vi "Adaptive Drain.vi"(0 "GEA2 Reference In":refnum<k24>, 1 "TC":dbl=1.2 format="%#_13g", 2 "H":dbl=5.0, 5 "BC":dbl=15.9 format="%#_13g", 7 "FC":dbl=-0.9 format="%#_13g", 9 "AD Timeout (s)":dbl=360.0 format="%#_13g", 11 "Error In":errorcluster, 12 "Pressure Threshold (Inchesx1000)":string="500") -> (3 "Actual Drain Time":dbl, 4 "GEA2 Reference Out":refnum<k24>, 6 "Pass/Fail?":bool, 10 "Report Text":string, 14 "Calculated Drain Time":dbl, 15 "Error Out":errorcluster)   [LabVIEW 2016, in "TLMB.lvlib"]
uses:
  Projects/TLMB.lvlib
  Q:/Common/DLLs/GEA3/GeaCommunication.dll
  Common/DLLs/GEA3/GeaCommunication.dll
  Common/LabVIEW GEA2 Toolkit/LabVIEW_GEA2_Toolkit.lvlibp/type defs/Source_Destination.ctl
  Common/LabVIEW GEA2 Toolkit/LabVIEW_GEA2_Toolkit.lvlibp/type defs/ERD Read Data In.ctl
  Common/LabVIEW GEA2 Toolkit/LabVIEW_GEA2_Toolkit.lvlibp/type defs/Data Type.ctl
  Common/LabVIEW GEA2 Toolkit/LabVIEW_GEA2_Toolkit.lvlibp
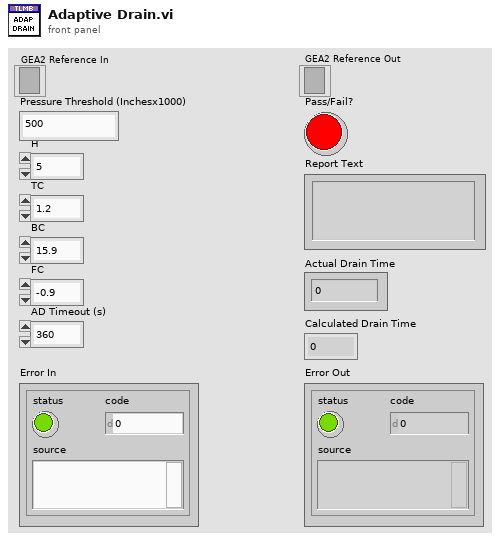
[diagram p1: front panel]
types:
  T1 = enum16{"EQ (==)", "NE (!=)", "GT (>)", "LT (<)", "GE (>=)", "LE (<=)", "GTLT(> <)", "GELE (>= <=)", "GELT (>= <)", "GTLE (> <=)", "LTGT (< >)", "LEGE (<= >=)", "LEGT (<= >)", "LTGE (< >=)", "No Comparison"}
  T2 = typedef "LabVIEW_GEA2_Toolkit.lvlibp/ERD Read Data In.ctl" = cluster{"ERD Number":u16, "Data Type":T3}
  T3 = typedef "LabVIEW_GEA2_Toolkit.lvlibp/Data Type.ctl" = enum16{"string", "boolean", "uint8_t", "uint16_t", "uint32_t", "uint64_t", "int8_t", "int16_t", "int32_t", "int64_t"}
  T4 = typedef "LabVIEW_GEA2_Toolkit.lvlibp/Source_Destination.ctl" = cluster{"Source":u8, "Destination":u8}
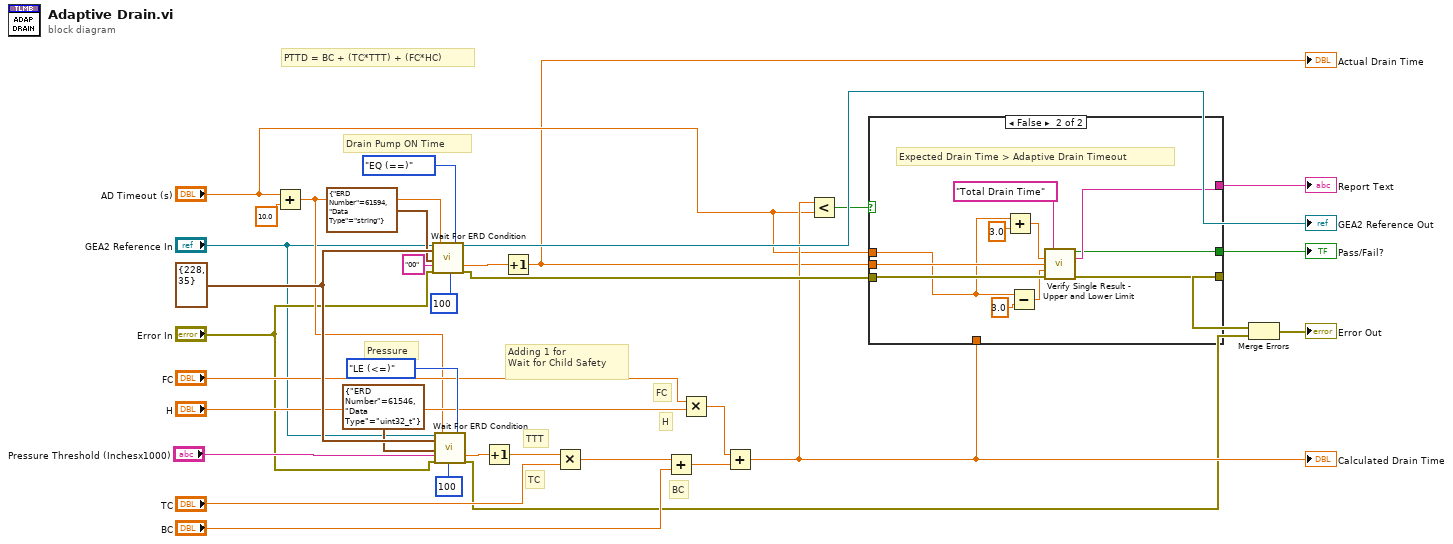
[diagram p0: block diagram]
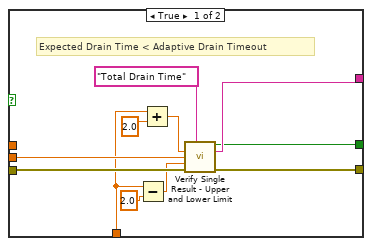
[diagram p2: hidden frame]
diagram:
  w34 = T4 {"Source"=228, "Destination"=35} ("GEA Inputs")
  # "Drain Pump ON Time"
  # "Pressure"
  # "Adding 1 for \nWait for Child Safety"
  # "H"
  # "FC"
  # "TTT"
  # "TC"
  # "BC"
  # "PTTD = BC + (TC*TTT) + (FC*HC)"
  n1 = Add(x="AD Timeout (s)", y=10.0) -> (x+y=w10:dbl)
  n2 = call "Wait For ERD Condition.vi"("GEA2 Reference In"="GEA2 Reference In", "GEA Inputs"=w34, "ERD Read Data"=T2 {"ERD Number"=61594, "Data Type"=enum."string"}, "Expected Low"="00", "Error In"="Error In", "Timeout (s)"=w10, "Loop Rate (ms)"=u32 100, "Comparison"=T1."EQ (==)") -> ("GEA2 Reference Out"=→"GEA2 Reference Out":refnum<k24>, "Execution Time"=w17:dbl, "Error Out"=w18:errorcluster)  [unwired: 7 in, 2 out]
  n3 = call "Wait For ERD Condition.vi"("GEA2 Reference In"="GEA2 Reference In", "GEA Inputs"=w34, "ERD Read Data"=T2 {"ERD Number"=61546, "Data Type"=enum."uint32_t"}, "Expected Low"="Pressure Threshold (Inchesx1000)", "Error In"="Error In", "Timeout (s)"=w10, "Loop Rate (ms)"=u32 100, "Comparison"=T1."LE (<=)") -> ("Execution Time"=w26:dbl, "Error Out"=w5:errorcluster)  [unwired: 7 in, 3 out]
  n4 = Increment(x=w26) -> (x+1=w23:dbl)
  n5 = Increment(x=w17) -> (x+1=w1:dbl)
  "Actual Drain Time" <- w1
  n6 = Multiply(x=w23, y="TC") -> (x*y=w22:dbl)
  n7 = Add(x=w22, y="BC") -> (x+y=w20:dbl)
  n8 = Multiply(x="FC", y="H") -> (x*y=w19:dbl)
  n9 = Add(x=w19, y=w20) -> (x+y=w9:dbl)
  "Calculated Drain Time" <- w9
  n10 = Less?(x=w9, y="AD Timeout (s)") -> (x < y?=w8:bool)
  n11 = case shown="False" w8 {
    tunnel: w1 -> [w45 w56]
    tunnel: w9 -> [w36 _]
    tunnel: w18 -> [w44 w55]
    tunnel: [w43 w54] -> w4
    tunnel: [w40 w51] -> w16
    tunnel: [w39 w50] -> w15
    tunnel: "AD Timeout (s)" -> [_ w47]
    frame True {
      # "Expected Drain Time < Adaptive Drain Timeout"
      n12 = Subtract(x=w36, y=2.0) -> (x-y=w41:dbl)
      n13 = Add(x=w36, y=2.0) -> (x+y=w42:dbl)
      n14 = call "Verify Single Result - Upper and Lower Limit.vi"("Name"="Total Drain Time", "Upper Limit"=w42, "Value"=w45, "Lower Limit"=w41, "Error In"=w44) -> ("Pass/Fail?"=w39:bool, "Report Text"=w40:string, "Error Out"=w43:errorcluster)  [unwired: 8 in]
    }
    frame False {
      # "Expected Drain Time > Adaptive Drain Timeout"
      n15 = Add(x=w47, y=3.0) -> (x+y=w53:dbl)
      n16 = Subtract(x=w47, y=3.0) -> (x-y=w52:dbl)
      n17 = call "Verify Single Result - Upper and Lower Limit.vi"("Name"="Total Drain Time", "Upper Limit"=w53, "Value"=w56, "Lower Limit"=w52, "Error In"=w55) -> ("Pass/Fail?"=w50:bool, "Report Text"=w51:string, "Error Out"=w54:errorcluster)  [unwired: 8 in]
    }
  }
  "Report Text" <- w16
  "Pass/Fail?" <- w15
  n18 = Merge Errors(w4, w5) -> (→"Error Out":errorcluster)
